vi "Create Live Random Data (Star).vi"(2 "Common Input Cluster":T2={"Input AnchorArray"=[], "DistanceLimitAnchor"=150.0, "Position Estimation Method"=0, "Max V variatie"=10.0, "Max h variatie"=30.0, "Enable error margin"=TRUE, "Error margin"=2} {"Max h variatie" format="%#_13g"; "Max V variatie" format="%#_13g"; "Position Estimation Method" items=["Star Configuration", "Swarm Method"]}, 3 "Tag.lvclass":refnum<class "Tag.lvclass">, 4 "error in (no error)":errorcluster, 5 "StarInput":T4) -> (6 "Star Configuration Indicators Cluster":T1, 8 "error IO":errorcluster)   [LabVIEW 2014]
doc: "This VI create random generated data based on its previous input, an array of Anchor objects and a single Tag object which we want its position estimated. The VI returns the Tag id, estimated position, and the altered array of Anchor objects. DistanceLimit control manages the limit on measured distances. If the measured distance >= DistanceLimit the distance is set to an invalid number so it will not be taken into account for position estimation. This control serves to simulate real world scenario where a signal can be lost\nafter a certain amount of meters."
uses:
  Tag.lvclass
  Anchor/Anchor.lvclass
  Position.lvclass
panel:
  out "Enable error margin":bool
  out "DistanceLimitAnchor":dbl
  out "Error margin":i32
  out "Input AnchorArray":refnum<class "Anchor.lvclass">[](array[class])
  out "Tag out":refnum<class "Tag.lvclass">
  out "AnchorIDDistanceCluster":T3
  out "NumberOfAnchors":i32
  out "AnchorClusterArray":T5(array[cluster])
  out "TagY":dbl
  out "TagX":dbl
  out "TagID":dbl
  out "x rand":dbl
  out "y rand":dbl
  out "Start y":dbl=30.0
  out "Start x":dbl=61.0
  # "Common Controls"
  # "Star Configuration Controls"
  # "Star Configuration Indicators"
  # "Error Indicator"
  # "Error Control"
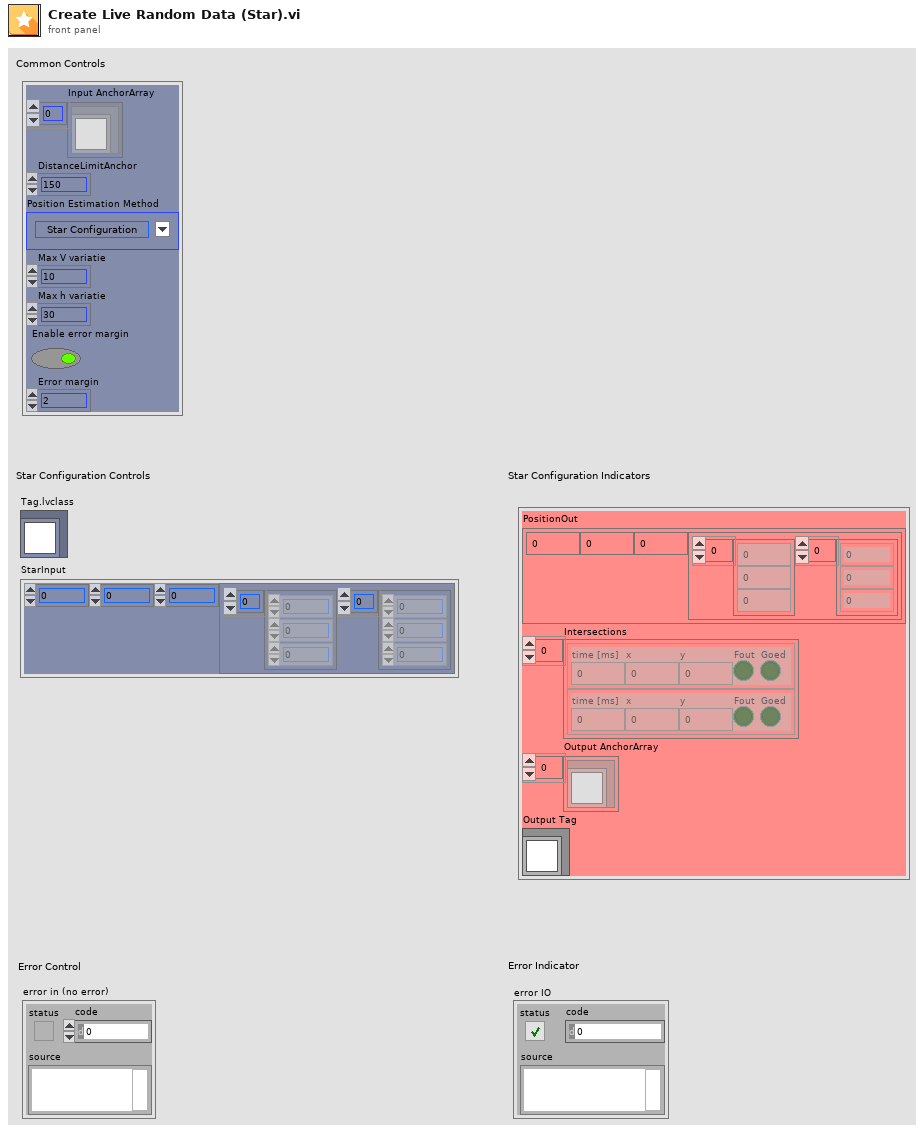
[diagram p1: front panel]
types:
  T1 = cluster{"PositionOut":cluster{"tagID":dbl, "EstimatedX":dbl, "EstimatedY":dbl, "anchorIDDistanceCluster":cluster{"anchorIDArray":dbl[], "anchorDistanceArray":dbl[]}}, "Intersections":cluster{"time [ms]":dbl, "x":dbl, "y":dbl, "Fout":bool, "Goed":bool}[], "Output AnchorArray":refnum<class "Anchor.lvclass">[], "Output Tag":refnum<class "Tag.lvclass">}
  T2 = cluster{"Input AnchorArray":refnum<class "Anchor.lvclass">[], "DistanceLimitAnchor":dbl, "Position Estimation Method":u32, "Max V variatie":dbl, "Max h variatie":dbl, "Enable error margin":bool, "Error margin":i32}
  T3 = cluster{"AnchorIDArrayConstant":dbl[], "AnchorDistanceConstant":dbl[]}
  T4 = cluster{"Tag":dbl, "X":dbl, "Y":dbl, "AnchorIDDistanceCluster":cluster{"AnchorIDArray":dbl[], "AnchorDistancesArray":dbl[]}}
  T5 = cluster{"AnchorID":dbl, "AnchorX":dbl, "AnchorY":dbl}[]
  T6 = cluster{"time [ms]":dbl, "x":dbl, "y":dbl, "Fout":bool, "Goed":bool}[]
  T7 = cluster{"tagID":dbl, "X":dbl, "Y":dbl, "anchorIDDistanceCluster":cluster{"anchorIDArray":dbl[], "anchorDistanceArray":dbl[]}}
  T8 = cluster{"PositionCluster [tagID, x, y, anchorID, distances]":cluster{"tagID":dbl, "X":dbl, "Y":dbl, "anchorIDDistanceCluster":cluster{"anchorIDArray":dbl[], "anchorDistanceArray":dbl[]}}, "Intersections":cluster{"time [ms]":dbl, "x":dbl, "y":dbl, "Fout":bool, "Goed":bool}[], "Output AnchorArray":refnum<class "Anchor.lvclass">[], "Tag out":refnum<class "Tag.lvclass">}
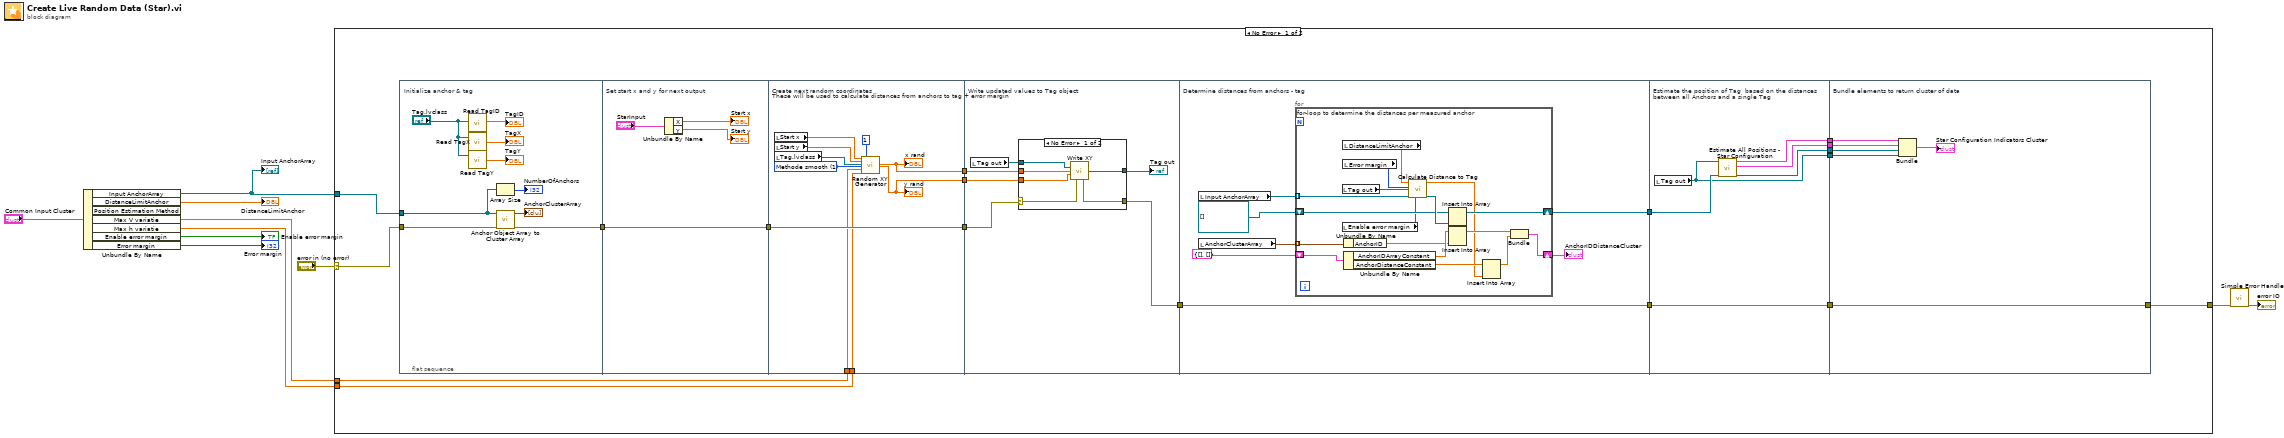
[diagram p0: block diagram]
diagram:
  n1 = Unbundle By Name("Common Input Cluster") -> ("Input AnchorArray"=w9:refnum<class "Anchor.lvclass">[], "DistanceLimitAnchor"=→"DistanceLimitAnchor":dbl, "Max V variatie"=w8:dbl, "Max h variatie"=w7:dbl, "Enable error margin"=→"Enable error margin":bool, "Error margin"=→"Error margin":i32)  [unwired: 1 out]
  "Input AnchorArray" <- w9
  n2 = case shown="No Error" "error in (no error)" {
    selector: "error in (no error)" -> [w26 w102]
    tunnel: w7 -> [w28 _]
    tunnel: w8 -> [w27 _]
    tunnel: [w25 w102] -> w3
    tunnel: w9 -> [w24 _]
    frame No Error {
      n3 = flat-sequence {
        tunnel: [w31] -> w23
        tunnel: w26 -> [w30]
        tunnel: w24 -> [w29]
        tunnel: [w38] -> w22
        tunnel: w23 -> [w38]
        tunnel: [w50] -> w21
        tunnel: [w49] -> w20
        tunnel: [w51] -> w19
        tunnel: w22 -> [w51]
        tunnel: w28 -> [w43]
        tunnel: w27 -> [w42]
        tunnel: w21 -> [w56]
        tunnel: w20 -> [w55]
        tunnel: w19 -> [w53]
        tunnel: [w52] -> w18
        tunnel: [w68] -> w17
        tunnel: w18 -> [w67]
        tunnel: [w67] -> w16
        tunnel: w17 -> [w95]
        tunnel: w16 -> [w94]
        tunnel: [w94] -> w15
        tunnel: [w93] -> w14
        tunnel: [w92] -> w13
        tunnel: [w91] -> w12
        tunnel: [w90] -> w11
        tunnel: [w101] -> w25
        tunnel: w15 -> [w101]
        tunnel: w14 -> [w99]
        tunnel: w13 -> [w98]
        tunnel: w12 -> [w97]
        tunnel: w11 -> [w96]
        frame #0 {
          # "Initialize anchor & tag"
          n4 = call "Read TagID.vi"("Tag in"="Tag.lvclass") -> ("TagID"=→"TagID":dbl)  [unwired: 16 in, 2 out]
          n5 = call-dynamic "Read TagX.vi"("Tag in"="Tag.lvclass") -> ("RealTagX"=→"TagX":dbl)  [unwired: 1 in, 2 out]
          n6 = call-dynamic "Read TagY.vi"("Tag in"="Tag.lvclass") -> ("RealTagY"=→"TagY":dbl)  [unwired: 1 in, 2 out]
          n7 = Array Size(array=w29) -> (size(s)=→"NumberOfAnchors":i32)
          n8 = call "Anchor Object Array to Cluster Array.vi"("error in (no error)"=w30, "AnchorArray In"=w29) -> ("error out"=w31:errorcluster, "AnchorArray Out"=→"AnchorClusterArray":T5)  [unwired: 8 in]
        }
        frame #1 {
          # "Set start x and y for next output"
          n9 = Unbundle By Name("StarInput") -> ("X"=→"Start x":dbl, "Y"=→"Start y":dbl)
        }
        frame #2 {
          w44 = u16 1 items=["Methode Random", "Methode smooth"] ("Random Methode")
          # "Create next random coordinates\nThese will be used to calculate distances from anchors to tag + error margin"
          n10 = local read "Start x"() -> (w47:dbl)
          n11 = local read "Start y"() -> (w46:dbl)
          n12 = local read "Tag.lvclass"() -> (w45:refnum<class "Tag.lvclass">)
          n13 = call "Random XY Generator.vi"("X start"=w47, "Y start"=w46, "Tag.lvclass"=w45, "Random Methode"=w44, "MaxVelocity"=w42, "MaxHeading"=w43, "number of rounds"=1) -> ("x"=w50:dbl, "y"=w49:dbl)  [unwired: 9 in, 2 out]
          "y rand" <- w49
          "x rand" <- w50
        }
        frame #3 {
          # "Write updated values to Tag object"
          n14 = local read "Tag out"() -> (w57:refnum<class "Tag.lvclass">)
          n15 = case shown="No Error" w53 {
            selector: w53 -> [w60 w65]
            tunnel: w57 -> [w63 w64]
            tunnel: w56 -> [w62 _]
            tunnel: w55 -> [w61 _]
            tunnel: [w59 w65] -> w52
            tunnel: [w58 w64] -> w54
            frame No Error {
              n16 = call "Write XY.vi"("Tag.lvclass"=w63, "TagX"=w62, "TagY"=w61, "error in (no error)"=w60) -> ("Tag Out"=w58:refnum<class "Tag.lvclass">, "error out"=w59:errorcluster)  [unwired: 10 in]
            }
            frame Error {
            }
          }
          "Tag out" <- w54
        }
        frame #4 {
          # "Determine distances from anchors - tag"
          n17 = local read "Input AnchorArray"() -> (w66:refnum<class "Anchor.lvclass">[])
          n18 = local read "AnchorClusterArray"() -> (w72:T5)
          n19 = for {
            tunnel: w72 -> [w89] mode=indexing
            shift-right: [w82] -> w70
            shift-left: T3 {"AnchorIDArrayConstant"=[], "AnchorDistanceConstant"=[]} ("AnchorIDDistanceClusterConstant") -> [w88]
            tunnel: w66 -> [w81] mode=indexing
            shift-right: [w78] -> w68
            shift-left: refnum<class "Anchor.lvclass">[] [] -> [w79]
            # "for-loop to determine the distances per measured anchor"
            n20 = local read "Tag out"() -> (w76:refnum<class "Tag.lvclass">)
            n21 = local read "Enable error margin"() -> (w73:bool)
            n22 = local read "DistanceLimitAnchor"() -> (w74:dbl)
            n23 = local read "Error margin"() -> (w75:i32)
            n24 = Unbundle By Name(w89) -> ("AnchorID"=w86:dbl)
            n25 = Unbundle By Name(w88) -> ("AnchorIDArrayConstant"=w87:dbl[], "AnchorDistanceConstant"=w85:dbl[])
            n26 = call "Calculate Distance to Tag.vi"("Enable error margin"=w73, "Anchor.lvclass In"=w81, "Tag.lvclass"=w76, "Error margin"=w75, "DistanceLimitAnchor"=w74) -> ("Anchor out"=w80:refnum<class "Anchor.lvclass">, "Distance"=w77:dbl)  [unwired: 5 in]
            n27 = Insert Into Array(array=w79, new element=w80) -> (w78:refnum<class "Anchor.lvclass">[])  [unwired: 1 in]
            n28 = Insert Into Array(array=w87, new element=w86) -> (w83:dbl[])  [unwired: 1 in]
            n29 = Insert Into Array(array=w85, new element=w77) -> (w84:dbl[])  [unwired: 1 in]
            n30 = Bundle("AnchorIDArrayConstant"=w83, "AnchorDistanceConstant"=w84) -> (w82:T3)  [unwired: 1 in]
          }
          "AnchorIDDistanceCluster" <- w70
        }
        frame #5 {
          # "Estimate the position of Tag  based on the distances between all Anchors and a single Tag"
          n31 = local read "Tag out"() -> (w90:refnum<class "Tag.lvclass">)
          n32 = call "Estimate All Positions - Star Configuration.vi"("Input AnchorArray"=w95, "Tag.lvclass"=w90) -> ("Output AnchorArray"=w91:refnum<class "Anchor.lvclass">[], "Intersections"=w92:T6, "PositionCluster [tagID, x, y, anchorID, distances]"=w93:T7)  [unwired: 7 in]
        }
        frame #6 {
          # "Bundle elements to return cluster of data"
          n33 = Bundle("PositionCluster [tagID, x, y, anchorID, distances]"=w99, "Intersections"=w98, "Output AnchorArray"=w97, "Tag out"=w96) -> (→"Star Configuration Indicators Cluster":T8)  [unwired: 1 in]
        }
      }
    }
    frame Error {
    }
  }
  n34 = call <vilib>:"Simple Error Handler.vi"("error in (no error)"=w3) -> ("error out"=→"error IO":errorcluster)  [unwired: 4 in, 4 out]
